vi "Receive Value Change Event.vi"(8 "error in (no error)":errorcluster, 10 "ValueChangeMsg":refnum<class "ValueChangeMsg.lvclass">, 11 "Main View In":refnum<class "Main View.lvclass">) -> (0 "error out":errorcluster, 3 "Main View Out":refnum<class "Main View.lvclass">)   [LabVIEW 2017, in "Main View.lvclass"]
doc: "<License>\nCopyright © 2017 Composed Systems, LLC | All rights reserved\nwww.composed.io\n\nAuthor: Ethan Stern <ethan.stern@composed.io>\n\nThis software is provided \"AS IS\" WITHOUT WARRANTIES, either express or implied, AND IS FOR EDUCATIONAL PURPOSES ONLY.\n</License>"
uses:
  <vilib>/gpm_packages/@cs/popup-viewmanager/Example/Main View/Main View.lvclass
  C:/Program Files/National Instruments/LabVIEW 2017/vi.lib/ActorFramework/Actor/Actor.lvclass
  <vilib>/gpm_packages/@cs/mva-viewable/Source/ActorEvents/IEventAggregator Messages/ValueChangeMsg/ValueChangeMsg.lvclass
  <vilib>/gpm_packages/@cs/mva-viewable/Source/ActorEvents/IEventAggregator Messages/ValueChangeMsg/ValueChangeMsg.lvclass/ValueChangeMsg.ctl
  <vilib>/ActorFramework/Actor/Actor.lvclass/Actor.ctl
  <vilib>/ActorFramework/Message Enqueuer/Message Enqueuer.lvclass/Message Enqueuer.ctl
  <vilib>/gpm_packages/@cs/popup-viewmanager/Example/Main View/Main View.lvclass/Main View.ctl
  <vilib>/gpm_packages/@cs/mva-dialogbox/source/DialogBoxViewManager/DialogBoxViewManager Messages/Launch Dialog Box Msg/Launch Dialog Box Msg.lvclass/Launch Dialog Box Msg.ctl
  <vilib>/ActorFramework/Message Enqueuer/Init from Existing Queue.vi
  <vilib>/ActorFramework/Message Enqueuer/Enqueue.vi
  <vilib>/gpm_packages/@cs/popup-viewmanager/Source/Popup ViewManager/Popup ViewManager.lvclass
  C:/Program Files/National Instruments/LabVIEW 2017/vi.lib/gpm_packages/@cs/mva-dialogbox/source/IDialogBox/IDialogBox/IDialogBox.lvclass
  <vilib>/gpm_packages/@cs/mva-dialogbox/source/DialogBoxViewManager/DialogBoxViewManager Messages/Launch Dialog Box Msg/Launch Dialog Box Msg.lvclass
  C:/Program Files/National Instruments/LabVIEW 2017/vi.lib/ActorFramework/Message/Message.lvclass
  <vilib>/ActorFramework/Message Priority Queue/Priority Enqueue.vi
  <vilib>/ActorFramework/Message Enqueuer/Message Enqueuer.lvclass
  <vilib>/gpm_packages/@cs/mva-dialogbox/source/DialogBoxViewManager/DialogBoxViewManager/DialogBoxViewManager.lvclass
  <vilib>/ActorFramework/Actor/Actor.lvclass
panel:
  out "error out 2":errorcluster
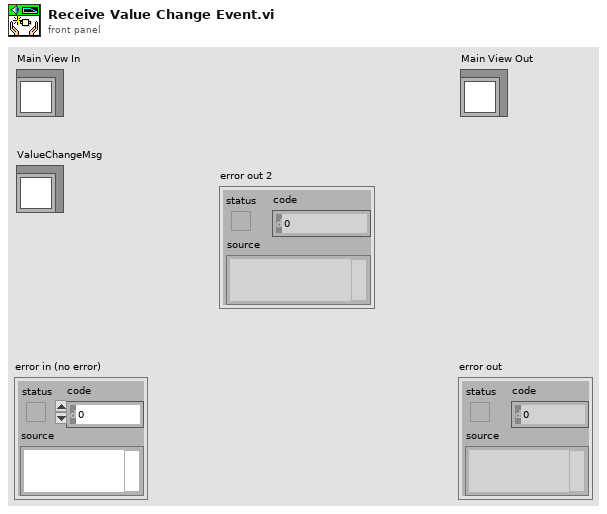
[diagram p1: front panel]
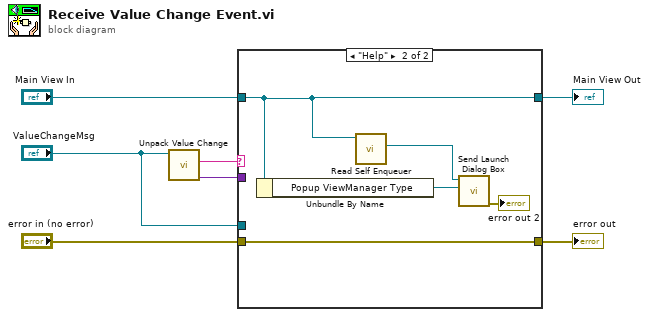
[diagram p0: block diagram]
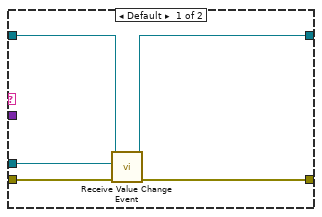
[diagram p2: hidden frame]
diagram:
  n1 = call <vilib>:"Unpack Value Change.vi"("ValueChangeMsg"="ValueChangeMsg") -> ("New Value"=w1:variant, "Control Label"=w2:string)  [unwired: 6 in, 3 out]
  n2 = case shown="\"Help\"" w2 {
    tunnel: [w12 w17] -> w7
    tunnel: [w11 w16] -> w6
    tunnel: "error in (no error)" -> [w10 w17]
    tunnel: "Main View In" -> [w9 w16]
    tunnel: "ValueChangeMsg" -> [w8 _]
    tunnel: w1 -> [_ _]
    frame Default {
      n3 = call-parent "Receive Value Change Event.vi"("error in (no error)"=w10, "ValueChangeMsg"=w8, "IViewable In"=w9) -> ("error out"=w12:errorcluster, "IViewable Out"=w11:refnum<class "Main View.lvclass">)  [unwired: 7 in]
    }
    frame "Help" {
      n4 = Unbundle By Name(w16) -> ("Popup ViewManager Type"=w14:refnum<class "Popup ViewManager.lvclass">)
      n5 = call <vilib>:"Read Self Enqueuer.vi"("Actor"=w16) -> ("Self Enqueuer"=w15:refnum<class "Message Enqueuer.lvclass">)  [unwired: 10 in]
      n6 = call <vilib>:"Send Launch Dialog Box.vi"("DialogBox"=w14, "Message Enqueuer"=w15) -> ("error out"=→"error out 2":errorcluster)  [unwired: 8 in, 1 out]
    }
  }
  "error out" <- w7
  "Main View Out" <- w6
